vi "Bernoulli Random.vi"(6 "seed":i32=-1, 7 "reset":bool, 9 "p":dbl=0.2, 11 "samples":i32=128) -> (0 "error":i32, 3 "Bernoulli random numbers":u32[](array[numeric]))   [LabVIEW 2020, in "NI_Gmath.lvlib"]
doc: "Generates random values from a variate X, where X describes the selected distribution type. You must manually select the polymorphic instance to use."
uses:
  NI_Gmath.lvlib
  NI_AALBase.lvlib
panel:
  # "Bernoulli Random"
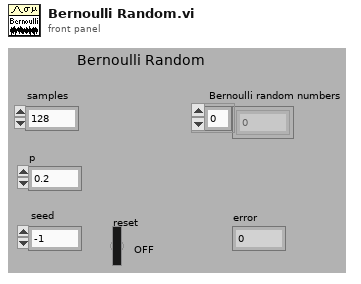
[diagram p1: front panel]
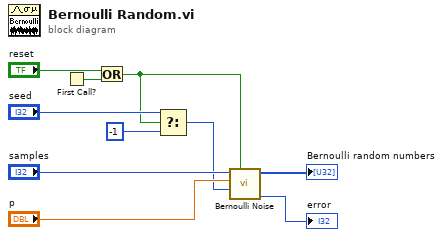
[diagram p0: block diagram]
diagram:
  n1 = First Call?() -> (First Call?: T/F=w6:bool)
  n2 = Or(x="reset", y=w6) -> (x .or. y?=w1:bool)
  n3 = Select(t="seed", s=w1, f=-1) -> (s? t:f=w2:i32)
  n4 = call "Bernoulli Noise.vi"("initialize?"=w1, "seed"=w2, "ones probability"="p", "samples"="samples") -> ("error"=→"error":i32, "bernoulli noise"=→"Bernoulli random numbers":u8[])  [unwired: 6 in]
